vi "Append Header.vi"(8 "error in (no error)":errorcluster, 9 "Paragraph.Style":refnum<class "Style.lvclass">, 10 "Paragraph.Text":string, 11 "xwpfDocument in":refnum<class "xwpfDocument.lvclass">) -> (0 "error out":errorcluster, 3 "xwpfDocument out":refnum<class "xwpfDocument.lvclass">)   [LabVIEW 2017, in "Word_Specific.lvlib" / "xwpfDocument.lvclass"]
uses:
  xwpfDocument.lvclass
  Styles/Style/Style.lvclass
  xwpfDocument.lvclass/xwpfDocument.ctl
  C:/Users/Neo/Desktop/Dev_Tools_BR/LabVIEW_NPOI/lib/NPOI 2.1.1/NPOI.OOXML.dll
  lib/NPOI 2.1.1/NPOI.OOXML.dll
panel:
  out "Text":string
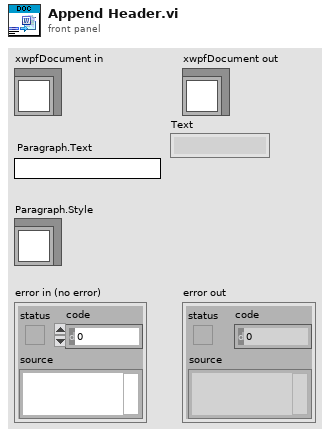
[diagram p1: front panel]
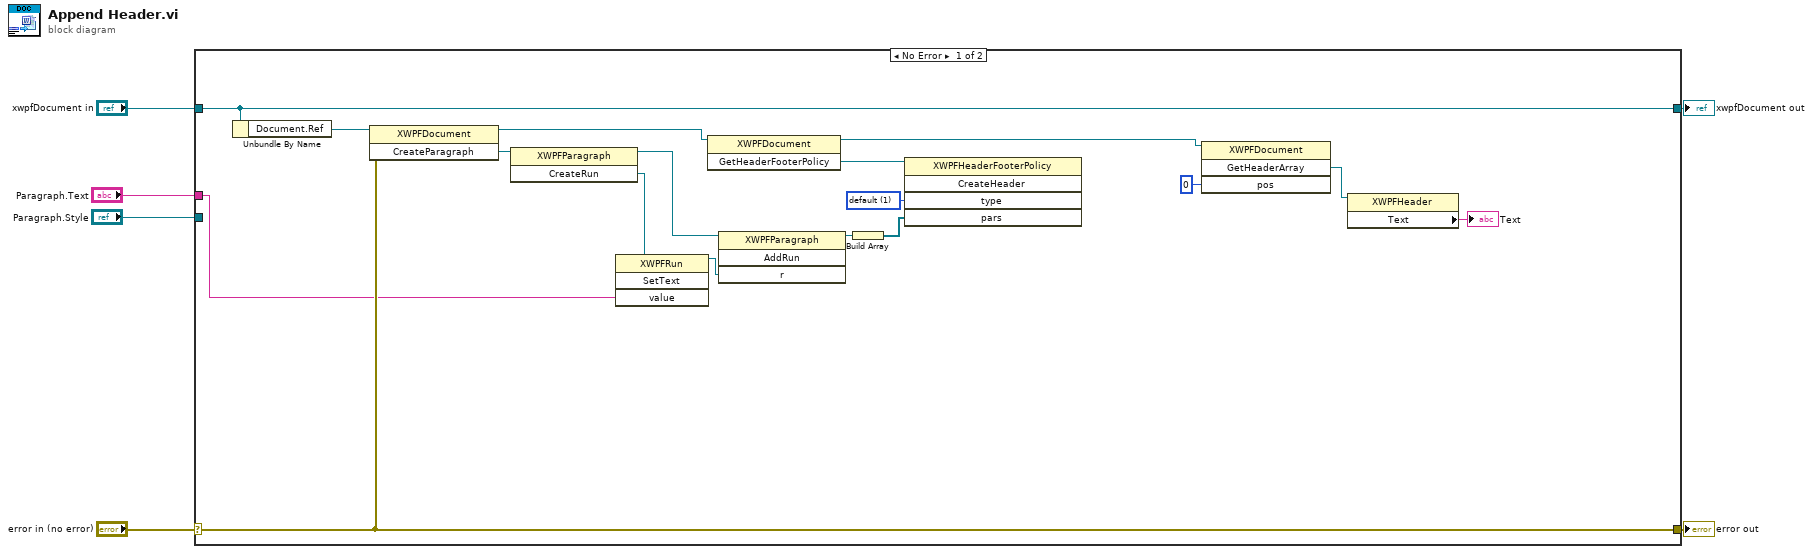
[diagram p0: block diagram]
diagram:
  n1 = case shown="No Error" "error in (no error)" {
    selector: "error in (no error)" -> [w18 w25]
    tunnel: [w18 w25] -> w6
    tunnel: [w22 w24] -> w4
    tunnel: "xwpfDocument in" -> [w22 w24]
    tunnel: "Paragraph.Text" -> [w15 _]
    tunnel: "Paragraph.Style" -> [_ _]
    frame No Error {
      w19 = 1 items=["even", "default", "first"] ("type")
      n2 = Unbundle By Name(w22) -> ("Document.Ref"=w23:refnum<k24>)
      n3 = invoke class="XWPFDocument" method="CreateParagraph"(reference=w23, error in=w18) -> (reference out=w21:refnum<k24>, "CreateParagraph"=w17:refnum<k24>)  [unwired: 1 in, 1 out]
      n4 = invoke class="XWPFParagraph" method="CreateRun"(reference=w17) -> (reference out=w7:refnum<k24>, "CreateRun"=w16:refnum<k24>)  [unwired: 2 in, 1 out]
      n5 = invoke class="XWPFRun" method="SetText"(reference=w16, "value"=w15) -> (reference out=w14:refnum<k24>)  [unwired: 2 in, 3 out]
      n6 = invoke class="XWPFDocument" method="GetHeaderFooterPolicy"(reference=w21) -> (reference out=w11:refnum<k24>, "GetHeaderFooterPolicy"=w20:refnum<k24>)  [unwired: 2 in, 1 out]
      n7 = invoke class="XWPFParagraph" method="AddRun"(reference=w7, "r"=w14) -> (reference out=w13:refnum<k24>)  [unwired: 2 in, 3 out]
      n8 = Build Array(w13) -> (w12:refnum<k24>[])
      n9 = invoke class="XWPFHeaderFooterPolicy" method="CreateHeader"(reference=w20, "type"=w19, "pars"=w12) -> ()  [unwired: 2 in, 5 out]
      n10 = invoke class="XWPFDocument" method="GetHeaderArray"(reference=w11, "pos"=0) -> ("GetHeaderArray"=w9:refnum<k24>)  [unwired: 2 in, 3 out]
      n11 = property class="XWPFHeader"(reference=w9) -> ("Text"=→"Text":string)  [unwired: 1 in, 2 out]
    }
    frame Error {
    }
  }
  "error out" <- w6
  "xwpfDocument out" <- w4
